vi "Main.vi"() -> ()   [LabVIEW 2019]
doc: "This template is for the Queued Message Handler design pattern.\n\nThe Event Handling Loop generates messages based on user interface actions.\n\nThe Message Handling Loop processes messages generated by the Event Handling Loop, or by other messages. The messages are string values, so new messages can be added easily to the Message Cases case structure in the Message Handling Loop. Each message cluster can also provide an optional value for Message Data, which is a variant that can be converted to whatever message-specific data is required."
uses:
  controls/UI Data.ctl
  support/Message Queue/Enqueue Message (Single).vi
  <vilib>/Utility/error.llb/Error Cluster From Error Code.vi
  <vilib>/ErrorRing/Error Ring.xnode
  support/Message Queue/Message Queue.lvlib
  support/User Event - Stop/User Event - Stop.lvlib
panel:
  in  "Finish":bool
  in  "Restart":bool
  out "Progress":u8(slide) scale=0.0..12.0
  in  "Convert":bool
  out "Tab Control":T1(tab)
  in  "Load File":bool
  in  "Number of Pole Pairs":dbl
  in  "D-Q Transform Angle":dbl
  in  "Phase A Resistance":dbl
  in  "Resistance A unit":enum16{"Ohms", "mOhms", "uOhms"}(ring)
  in  "Phase B Resistance":dbl
  in  "Resistance B unit":enum16{"Ohms", "mOhms", "uOhms"}(ring)
  in  "Phase C Resistance":dbl
  in  "Resistance C unit":enum16{"Ohms", "mOhms", "uOhms"}(ring)
  in  "Direct Current (Id)":dbl[](array[numeric])
  in  "Id unit":enum16{"A", "mA"}(ring)
  in  "Quadratic Current (Iq)":dbl[](array[numeric])
  in  "Iq unit":enum16{"A", "mA"}(ring)
  in  "Direct Inductance (Ld)":dbl[][](array[numeric])
  in  "Ld unit":enum16{"H", "mH", "uH"}(ring)
  in  "Quadratic Inductance (Lq)":dbl[][](array[numeric])
  in  "Lq unit":enum16{"H", "mH", "uH"}(ring)
  in  "Permanent Magnet Flux (Fm)":dbl[][](array[numeric])
  in  "Fm unit":enum16{"Wb", "mWb"}(ring)
  in  "Perm Magnet Flux Scalar":dbl caption="Permanet Magnet Flux (Fm)"
  out "Iq size":i32
  out "Id size":i32
  out "Status":string
  out "Ld":i32[](array[numeric])
  out "Fm":i32[](array[numeric])
  out "Lq":i32[](array[numeric])
  out "JSON File Path":path
  in  "Back":bool
  in  "Next":bool
  # "Step 1: Select the spreadsheet file containing the machine parameters and click Next once it is open."
  # "Step 2: Please fill in the field below with the Number of Poles Pairs OR copy it from the spreadsheet."
  # "Step 3: Please fill in the field below with the D-Q Transform Angle OR copy it from the spreadsheet. Leave it as 0 if you don't have this information."
  # "Step 4: Please fill in the field below with the Phase A Resistance OR copy it from the spreadsheet."
  # "Step 5: Please fill in the field below with the Phase B Resistance OR copy it from the spreadsheet."
  # "Step 6: Please fill in the field below with the Phase C Resistance OR copy it from the spreadsheet."
  # "Step 7: Please fill in the field below with the Current values along the Direct axis of the stator OR copy it from the spreadsheet."
  # "Unit:"
  # "Step 8: Please fill in the field below with the Current values along the Quadratic axis of the stator OR copy it from the spreadsheet."
  # "Unit:"
  # "Step 9: Please fill in the field below with the Direct Inductance OR copy it from the spreadsheet."
  # "Unit:"
  # "Step 10: Please fill in the field below with the Quadratic Inductance OR copy it from the spreadsheet."
  # "Unit:"
  # "Step 11: Please fill in the field below with the Permanent Magnet Flux OR copy it from the spreadsheet. NOTE: Fm parameter is accepted as a scalar or 2D-array."
  # "Unit:"
  # "Step 12: Model converted and saved in the following directory:"
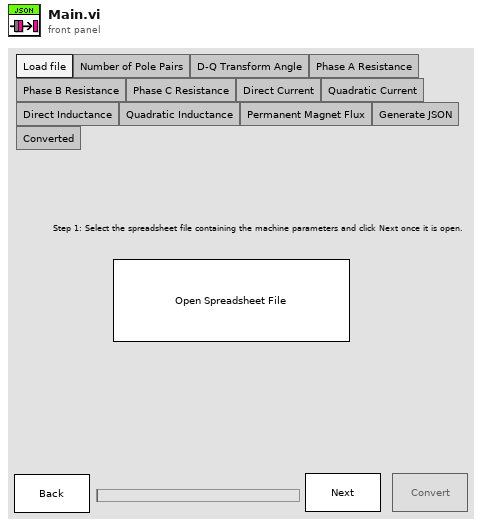
[diagram p1: front panel]
types:
  T1 = enum32{"Load file", "Number of Pole Pairs", "D-Q Transform Angle", "Phase A Resistance", "Phase B Resistance", "Phase C Resistance", "Direct Current", "Quadratic Current", "Direct Inductance", "Quadratic Inductance", "Permanent Magnet Flux", "Generate JSON", "Converted"}
  T2 = typedef "UI Data.ctl" = cluster{"Active tab":u32, "Next ref":refnum<vi>, "Back ref":refnum<vi>, "Convert ref":refnum<vi>, "Restart ref":refnum<vi>, "Finish ref":refnum<vi>, "selected path":path, "VDQ Model":cluster{"PolePairs":dbl, "DqTransformAngleOffset":dbl, "Ra":dbl, "Rb":dbl, "Rc":dbl, "Id_axis":dbl[], "Iq_axis":dbl[], "Ld":dbl[][], "Lq":dbl[][], "Fm":dbl[][]}, "saved path":path, "Scalar Fm ref":refnum<vi>, "2D Fm ref":refnum<vi>, "Current sorted?":cluster{"Id sorted?":bool, "Iq sorted?":bool}}
  T3 = typedef "Message Queue.lvlib/All Message Queues.ctl" = cluster{"UI":refnum<queue>}
  T4 = enum8{"Enabled", "Disabled", "Disabled and Grayed Out"}
  T5 = enum16{"open", "replace", "create", "open or create", "replace or create", "replace or create with confirmation"}
  T6 = cluster{"Id size":i32, "Iq size":i32, "Ld size":i32[], "Lq size":i32[], "FM size":i32[]}
  T7 = cluster{"PolePairs":dbl, "DqTransformAngleOffset":dbl, "Ra":dbl, "Rb":dbl, "Rc":dbl, "Id_axis":dbl[], "Iq_axis":dbl[], "Ld":dbl[][], "Lq":dbl[][], "Fm":dbl[][]}
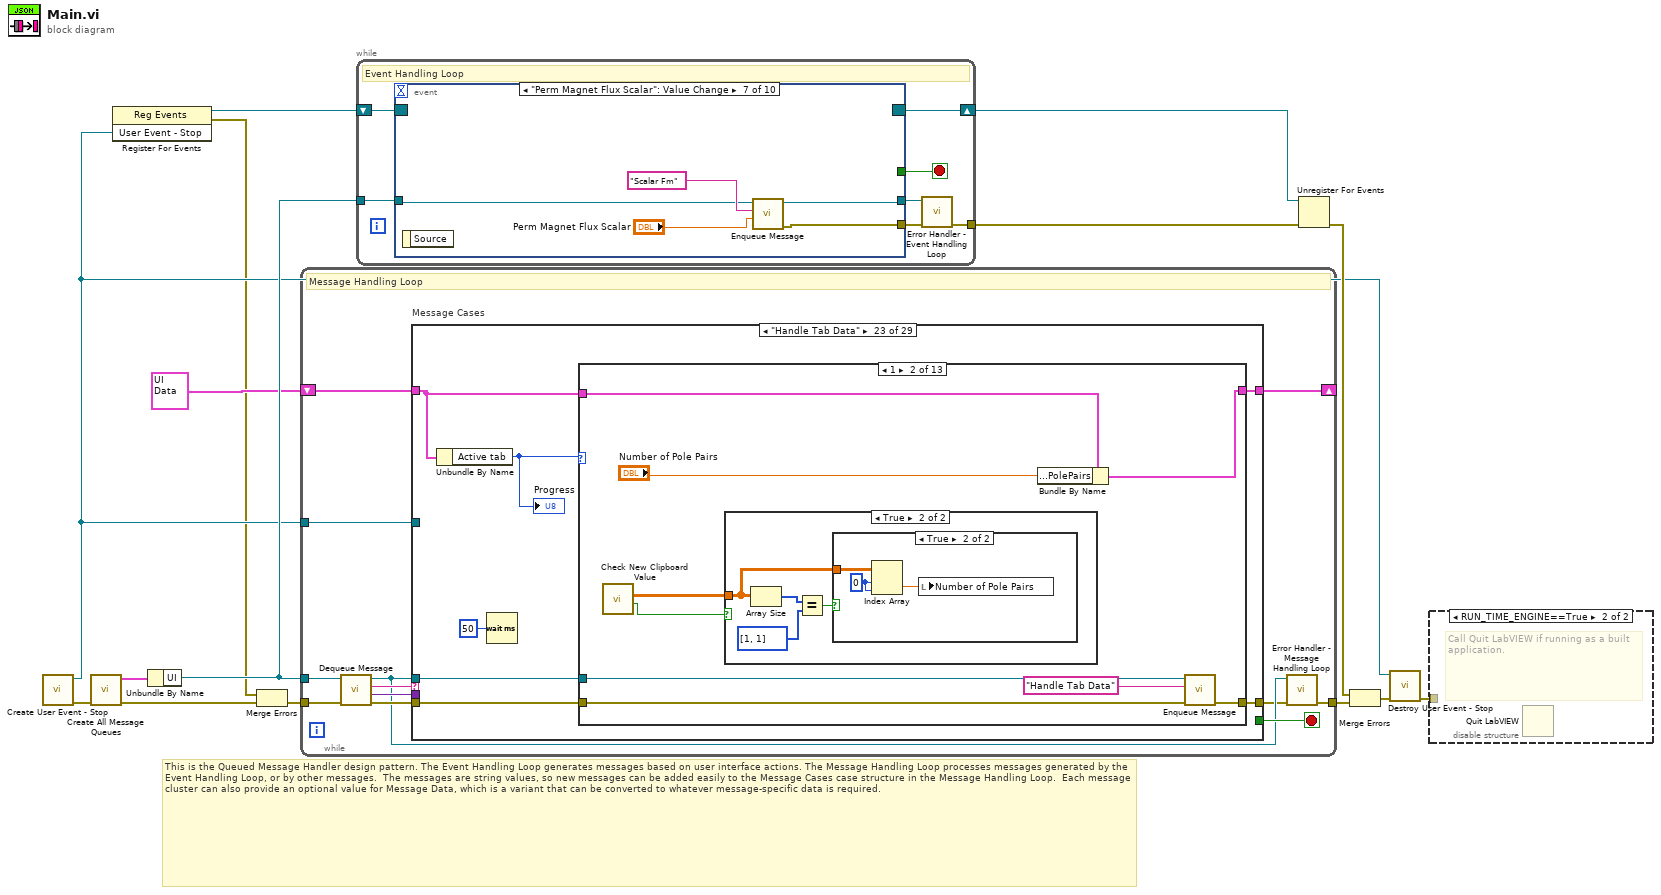
[diagram p0: block diagram]
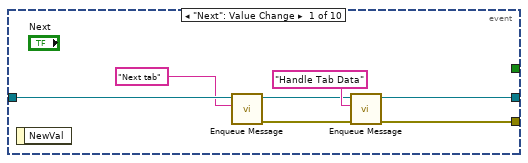
[diagram p3: hidden frame]
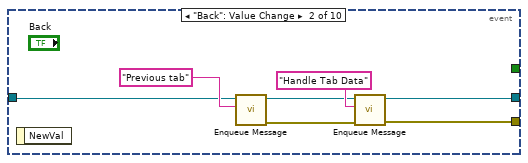
[diagram p4: hidden frame]
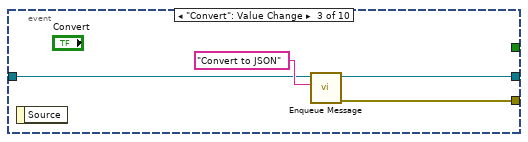
[diagram p5: hidden frame]
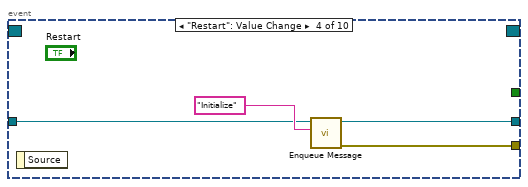
[diagram p6: hidden frame]
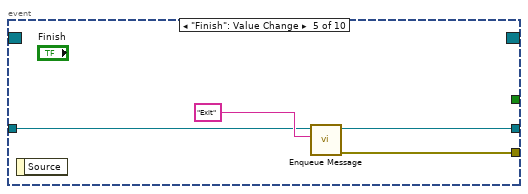
[diagram p7: hidden frame]
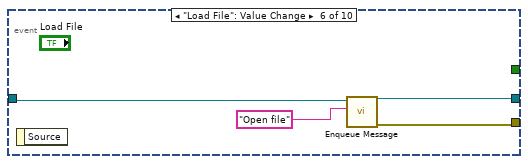
[diagram p8: hidden frame]
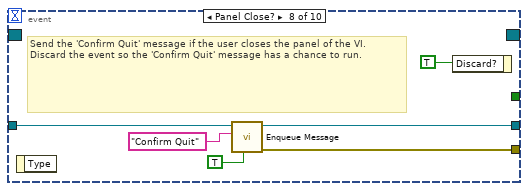
[diagram p9: hidden frame]
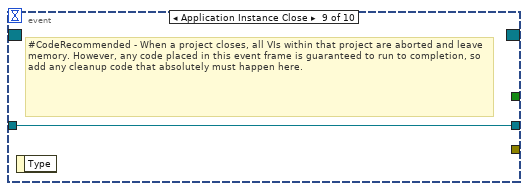
[diagram p10: hidden frame]
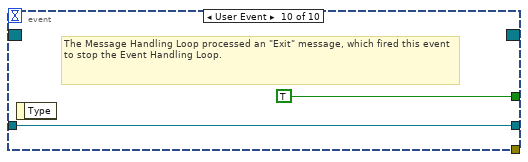
[diagram p11: hidden frame]
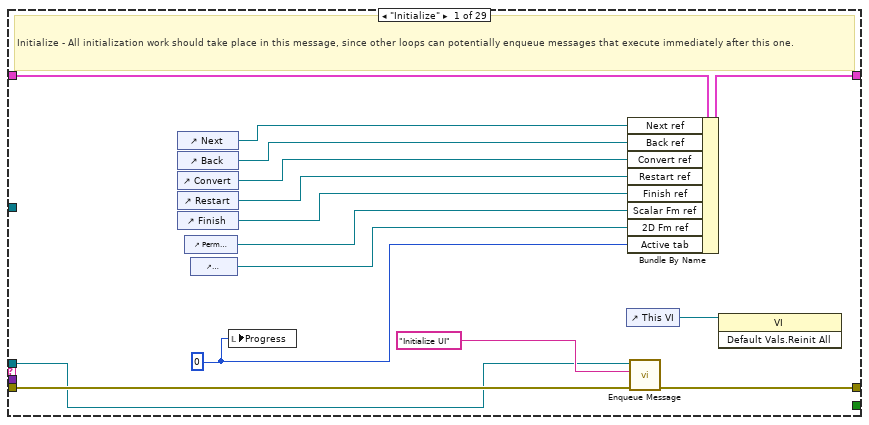
[diagram p12: hidden frame]
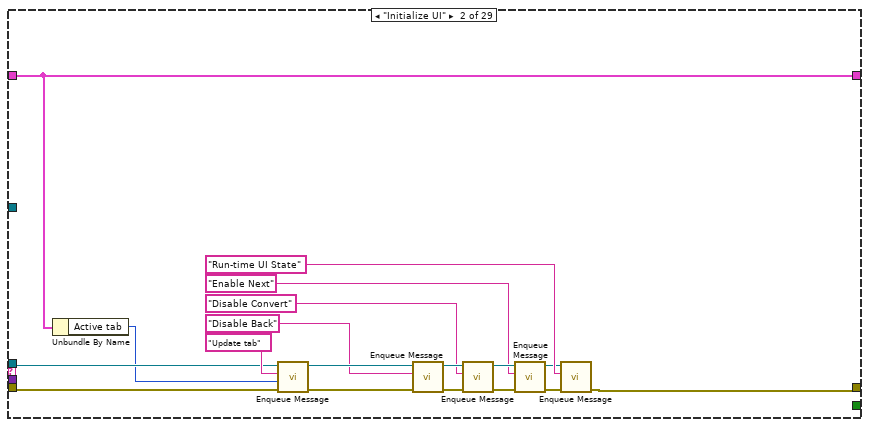
[diagram p13: hidden frame]
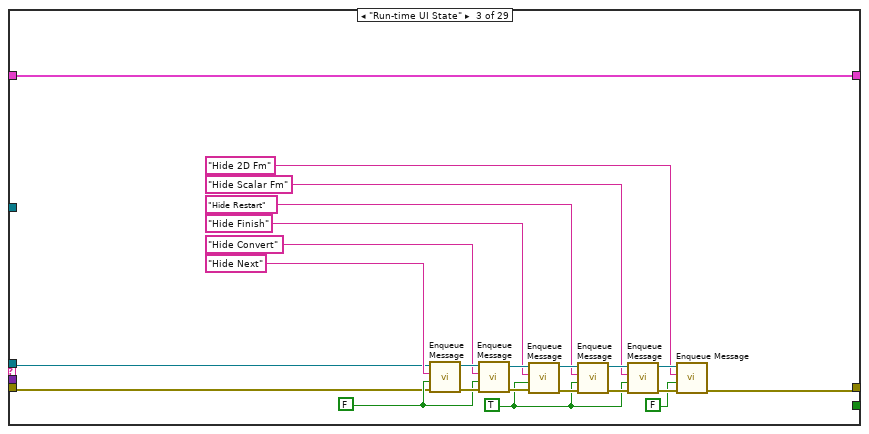
[diagram p14: hidden frame]
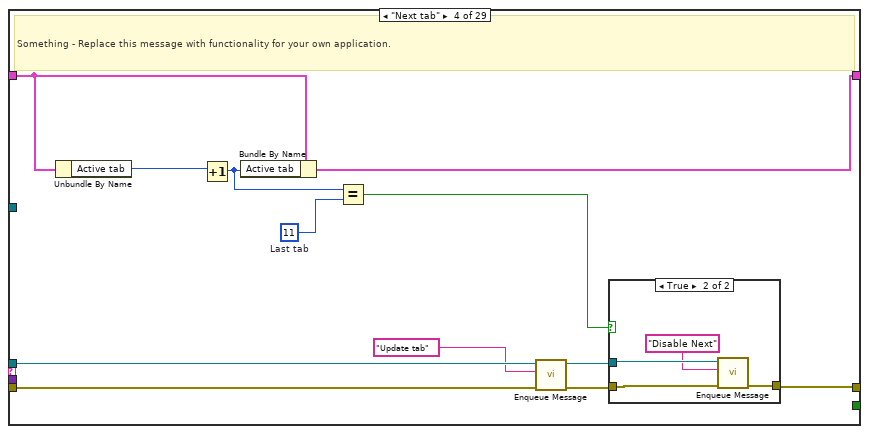
[diagram p15: hidden frame]
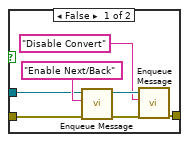
[diagram p16: hidden frame]
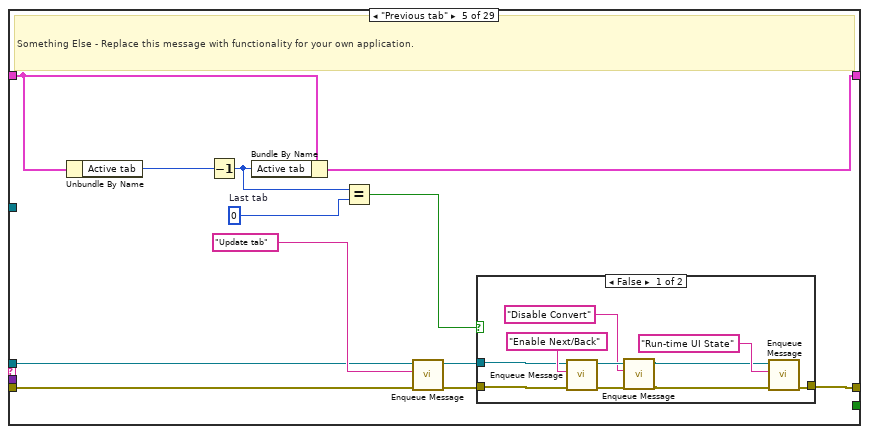
[diagram p17: hidden frame]
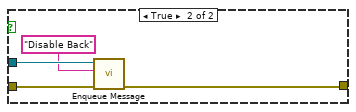
[diagram p18: hidden frame]
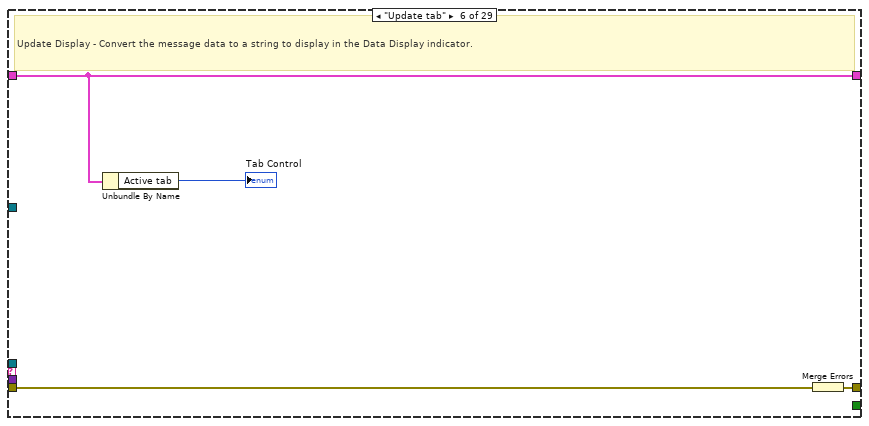
[diagram p19: hidden frame]
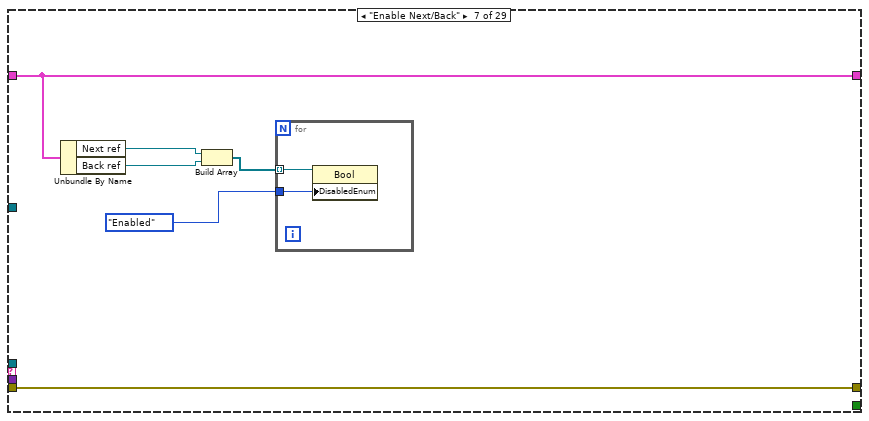
[diagram p20: hidden frame]
diagram:
  # "This is the Queued Message Handler design pattern. The Event Handling Loop generates messages based on user interface actions. The Message Handling Loop processes messages generated by the Event Handling Loop, or by other messages.  The messages are string values, so new messages can be added easily to the Message Cases case structure in the Message Handling Loop.  Each message cluster can also provide an optional value for Message Data, which is a variant that can be converted to whatever message-specific data is required."
  n1 = call "Create User Event - Stop.vi"() -> ("error out"=w11:errorcluster, "User Event - Stop"=w3:refnum<user-event>)  [unwired: 10 in]
  n2 = call "Create All Message Queues.vi"("error in (no error)"=w11) -> ("error out"=w15:errorcluster, "Message Queues out"=w14:T3)  [unwired: 9 in]
  n3 = register-events(w3) -> (reference out=w4:refnum<event-registration>, error out=w1:errorcluster)  [unwired: 2 in]
  n4 = Unbundle By Name(w14) -> ("UI"=w12:refnum<queue>)
  n5 = Merge Errors(w1, w15) -> (w2:errorcluster)
  n6 = while {
    tunnel: w12 -> [w19]
    shift-right: [w26] -> _
    shift-left: T2 {"Active tab"=0, "Next ref"=refnum, "Back ref"=refnum, "Convert ref"=refnum, "Restart ref"=refnum, "Finish ref"=refnum, "selected path"=path "", "VDQ Model"={"PolePairs"=0.0, "DqTransformAngleOffset"=0.0, "Ra"=0.0, "Rb"=0.0, "Rc"=0.0, "Id_axis"=[], "Iq_axis"=[], "Ld"=[], "Lq"=[], "Fm"=[]}, "saved path"=path "", "Scalar Fm ref"=refnum, "2D Fm ref"=refnum, "Current sorted?"={"Id sorted?"=FALSE, "Iq sorted?"=FALSE}} ("Data Cluster") -> [w27]
    tunnel: w3 -> [w24]
    tunnel: w2 -> [w23]
    tunnel: [w17] -> w13
    stop <- w25 stop-if-true
    # "Message Handling Loop"
    n7 = call "Dequeue Message.vi"("error in (no error)"=w23, "Message Queue"=w19) -> ("error out"=w22:errorcluster, "Message Data"=w20:variant, "Message"=w21:string, "dup Message Queue"=w18:refnum<queue>)  [unwired: 6 in]
    n8 = case "Message Cases" shown="\"Handle Tab Data\"" w21 {
      selector: w21 -> [_ _ _ _ _ _ _ _ _ _ _ _ _ _ _ _ _ _ _ _ _ _ _ _ _ _ _ _ w587]
      tunnel: w18 -> [w36 w49 w71 w94 w117 _ _ _ _ _ _ _ _ _ _ _ _ _ w223 _ _ _ w260 w531 _ w568 _ w586 _]
      tunnel: w22 -> [w42 w50 w70 w95 w116 w135 w142 w148 w152 w154 w159 w164 w170 w182 w191 w200 w209 w218 w222 w239 w247 w258 w264 w521 w565 w572 w575 w579 _]
      tunnel: [w31 w43 w66 w84 w108 w136 w142 w148 w152 w153 w158 w163 w172 w183 w192 w201 w210 w219 w224 w239 w246 w248 w265 w543 w559 w570 w573 w582 w588] -> w16
      tunnel: w27 -> [w41 w48 w83 w91 w115 w134 w141 w147 w151 w157 w162 w167 w176 w185 w194 w203 w212 w221 w237 w238 w244 w250 w262 w540 w564 w571 w574 w585 w589]
      tunnel: [w40 w48 w83 w90 w114 w134 w141 w147 w151 w157 w162 w167 w176 w185 w194 w203 w212 w221 w237 w238 w245 w250 w263 w539 w564 w571 w574 w585 w589] -> w26
      tunnel: [_ _ _ _ _ _ _ _ _ _ _ _ _ _ _ _ _ _ _ _ _ _ _ _ _ _ _ TRUE _] -> w25
      tunnel: w20 -> [_ _ _ _ _ _ _ _ _ _ _ _ w169 w179 w188 w197 w206 w215 _ _ _ w257 _ _ w563 _ _ w576 _]
      tunnel: w24 -> [_ _ _ _ _ _ _ _ _ _ _ _ _ _ _ _ _ _ _ _ _ _ _ _ _ _ _ w581 _]
      frame "Initialize" {
        w34 = u32 0
        # "Initialize - All initialization work should take place in this message, since other loops can potentially enqueue messages that execute immediately after this one."
        n9 = control-ref of="Next"() -> (w39:refnum<vi>)
        n10 = control-ref of="Back"() -> (w37:refnum<vi>)
        n11 = control-ref of="Convert"() -> (w35:refnum<vi>)
        n12 = control-ref of="Restart"() -> (w33:refnum<vi>)
        n13 = control-ref of="Finish"() -> (w32:refnum<vi>)
        n14 = control-ref of="Perm Magnet Flux Scalar"() -> (w29:refnum<vi>)
        n15 = control-ref of="Permanent Magnet Flux (Fm)"() -> (w28:refnum<vi>)
        n16 = local write "Progress"(w34) -> ()
        n17 = control-ref of="This VI"() -> (w30:refnum<vi>)
        n18 = Bundle By Name(cluster=w41, "Next ref"=w39, "Back ref"=w37, "Convert ref"=w35, "Restart ref"=w33, "Finish ref"=w32, "Scalar Fm ref"=w29, "2D Fm ref"=w28, "Active tab"=w34) -> (w40:T2)
        n19 = call-poly "Enqueue Message.vi"("error in (no error)"=w42, "Message"="Initialize UI", "Message Queue"=w36) -> ("error out"=w31:errorcluster)  [unwired: 7 in, 1 out]
        n20 = invoke class="VI" method="Default Vals.Reinit All"(reference=w30) -> ()  [unwired: 2 in, 3 out]
      }
      frame "Initialize UI" {
        n21 = Unbundle By Name(w48) -> ("Active tab"=w47:u32)
        n22 = call-poly "Enqueue Message.vi"("error in (no error)"=w50, "Message Data"=w47, "Message"="Update tab", "Message Queue"=w49) -> ("error out"=w60:errorcluster, "dup Message Queue"=w59:refnum<queue>)  [unwired: 6 in]
        n23 = call-poly "Enqueue Message.vi"("error in (no error)"=w60, "Message"="Disable Back", "Message Queue"=w59) -> ("error out"=w58:errorcluster, "dup Message Queue"=w57:refnum<queue>)  [unwired: 7 in]
        n24 = call-poly "Enqueue Message.vi"("error in (no error)"=w58, "Message"="Disable Convert", "Message Queue"=w57) -> ("error out"=w56:errorcluster, "dup Message Queue"=w55:refnum<queue>)  [unwired: 7 in]
        n25 = call-poly "Enqueue Message.vi"("error in (no error)"=w56, "Message"="Enable Next", "Message Queue"=w55) -> ("error out"=w44:errorcluster, "dup Message Queue"=w45:refnum<queue>)  [unwired: 7 in]
        n26 = call-poly "Enqueue Message.vi"("error in (no error)"=w44, "Message"="Run-time UI State", "Message Queue"=w45) -> ("error out"=w43:errorcluster)  [unwired: 7 in, 1 out]
      }
      frame "Run-time UI State" {
        w62 = TRUE
        w72 = FALSE
        n27 = call-poly "Enqueue Message.vi"("error in (no error)"=w70, "Message Data"=w72, "Message"="Hide Next", "Message Queue"=w71) -> ("error out"=w75:errorcluster, "dup Message Queue"=w81:refnum<queue>)  [unwired: 6 in]
        n28 = call-poly "Enqueue Message.vi"("error in (no error)"=w75, "Message Data"=w72, "Message"="Hide Convert", "Message Queue"=w81) -> ("error out"=w74:errorcluster, "dup Message Queue"=w80:refnum<queue>)  [unwired: 6 in]
        n29 = call-poly "Enqueue Message.vi"("error in (no error)"=w74, "Message Data"=w62, "Message"="Hide Finish", "Message Queue"=w80) -> ("error out"=w73:errorcluster, "dup Message Queue"=w79:refnum<queue>)  [unwired: 6 in]
        n30 = call-poly "Enqueue Message.vi"("error in (no error)"=w73, "Message Data"=w62, "Message"="Hide Restart", "Message Queue"=w79) -> ("error out"=w67:errorcluster, "dup Message Queue"=w65:refnum<queue>)  [unwired: 6 in]
        n31 = call-poly "Enqueue Message.vi"("error in (no error)"=w67, "Message Data"=w62, "Message"="Hide Scalar Fm", "Message Queue"=w65) -> ("error out"=w69:errorcluster, "dup Message Queue"=w68:refnum<queue>)  [unwired: 6 in]
        n32 = call-poly "Enqueue Message.vi"("error in (no error)"=w69, "Message Data"=FALSE, "Message"="Hide 2D Fm", "Message Queue"=w68) -> ("error out"=w66:errorcluster)  [unwired: 6 in, 1 out]
      }
      frame "Next tab" {
        w89 = u32 11  # Last tab
        # "Something - Replace this message with functionality for your own application."
        n33 = Unbundle By Name(w91) -> ("Active tab"=w92:u32)
        n34 = Increment(x=w92) -> (x+1=w88:u32)
        n35 = Bundle By Name(cluster=w91, "Active tab"=w88) -> (w90:T2)
        n36 = Equal?(x=w88, y=w89) -> (x = y?=w87:bool)
        n37 = call-poly "Enqueue Message.vi"("error in (no error)"=w95, "Message"="Update tab", "Message Queue"=w94) -> ("error out"=w86:errorcluster, "dup Message Queue"=w85:refnum<queue>)  [unwired: 7 in]
        n38 = case shown="True" w87 {
          tunnel: w86 -> [w101 w106]
          tunnel: w85 -> [w100 w104]
          tunnel: [w98 w105] -> w84
          frame False {
            n39 = call-poly "Enqueue Message.vi"("error in (no error)"=w101, "Message"="Enable Next/Back", "Message Queue"=w100) -> ("error out"=w99:errorcluster, "dup Message Queue"=w97:refnum<queue>)  [unwired: 7 in]
            n40 = call-poly "Enqueue Message.vi"("error in (no error)"=w99, "Message"="Disable Convert", "Message Queue"=w97) -> ("error out"=w98:errorcluster)  [unwired: 7 in, 1 out]
          }
          frame True {
            n41 = call-poly "Enqueue Message.vi"("error in (no error)"=w106, "Message"="Disable Next", "Message Queue"=w104) -> ("error out"=w105:errorcluster)  [unwired: 7 in, 1 out]
          }
        }
      }
      frame "Previous tab" {
        w112 = u32 0  # Last tab
        # "Something Else - Replace this message with functionality for your own application."
        n42 = Unbundle By Name(w115) -> ("Active tab"=w113:u32)
        n43 = Decrement(x=w113) -> (x-1=w107:u32)
        n44 = Bundle By Name(cluster=w115, "Active tab"=w107) -> (w114:T2)
        n45 = Equal?(x=w107, y=w112) -> (x = y?=w111:bool)
        n46 = call-poly "Enqueue Message.vi"("error in (no error)"=w116, "Message"="Update tab", "Message Queue"=w117) -> ("error out"=w110:errorcluster, "dup Message Queue"=w109:refnum<queue>)  [unwired: 7 in]
        n47 = case shown="False" w111 {
          tunnel: w110 -> [w124 w132]
          tunnel: w109 -> [w123 w131]
          tunnel: [w119 w129] -> w108
          frame False {
            n48 = call-poly "Enqueue Message.vi"("error in (no error)"=w124, "Message"="Enable Next/Back", "Message Queue"=w123) -> ("error out"=w127:errorcluster, "dup Message Queue"=w126:refnum<queue>)  [unwired: 7 in]
            n49 = call-poly "Enqueue Message.vi"("error in (no error)"=w127, "Message"="Disable Convert", "Message Queue"=w126) -> ("error out"=w120:errorcluster, "dup Message Queue"=w121:refnum<queue>)  [unwired: 7 in]
            n50 = call-poly "Enqueue Message.vi"("error in (no error)"=w120, "Message"="Run-time UI State", "Message Queue"=w121) -> ("error out"=w119:errorcluster)  [unwired: 7 in, 1 out]
          }
          frame True {
            n51 = call-poly "Enqueue Message.vi"("error in (no error)"=w132, "Message"="Disable Back", "Message Queue"=w131) -> ("error out"=w129:errorcluster)  [unwired: 7 in, 1 out]
          }
        }
      }
      frame "Update tab" {
        # "Update Display - Convert the message data to a string to display in the Data Display indicator."
        n52 = Unbundle By Name(w134) -> ("Active tab"=→"Tab Control":u32)
        n53 = Merge Errors(w135) -> (w136:errorcluster)
      }
      frame "Enable Next/Back" {
        n54 = Unbundle By Name(w141) -> ("Next ref"=w140:refnum<vi>, "Back ref"=w139:refnum<vi>)
        n55 = Build Array(w140, w139) -> (w138:refnum<vi>[])
        n56 = for {
          tunnel: w138 -> [w144] mode=indexing
          tunnel: T4."Enabled" ("Disabled") -> [w143]
          n57 = property class="Bool"(reference=w144, "DisabledEnum"=w143) -> ()  [unwired: 1 in, 2 out]
        }
      }
      frame "Enable Convert" {
        n58 = Unbundle By Name(w147) -> ("Convert ref"=w145:refnum<vi>)
        n59 = property class="Bool"(reference=w145, "DisabledEnum"=T4."Enabled" ("Disabled")) -> ()  [unwired: 1 in, 2 out]
      }
      frame "Enable Next" {
        n60 = Unbundle By Name(w151) -> ("Next ref"=w149:refnum<vi>)
        n61 = property class="Bool"(reference=w149, "DisabledEnum"=T4."Enabled" ("Disabled")) -> ()  [unwired: 1 in, 2 out]
      }
      frame "Disable Next" {
        n62 = Unbundle By Name(w157) -> ("Next ref"=w156:refnum<vi>)
        n63 = property class="Bool"(reference=w156, error in=w154, "DisabledEnum"=T4."Disabled and Grayed Out" ("Disabled")) -> (error out=w153:errorcluster)  [unwired: 1 out]
      }
      frame "Disable Back" {
        n64 = Unbundle By Name(w162) -> ("Back ref"=w161:refnum<vi>)
        n65 = property class="Bool"(reference=w161, error in=w159, "DisabledEnum"=T4."Disabled and Grayed Out" ("Disabled")) -> (error out=w158:errorcluster)  [unwired: 1 out]
      }
      frame "Disable Convert" {
        n66 = Unbundle By Name(w167) -> ("Convert ref"=w166:refnum<vi>)
        n67 = property class="Bool"(reference=w166, error in=w164, "DisabledEnum"=T4."Disabled and Grayed Out" ("Disabled")) -> (error out=w163:errorcluster)  [unwired: 1 out]
      }
      frame "Hide Next" {
        n68 = Variant To Data(error in=w170, type=FALSE ("Visible"), Variant=w169) -> (data=w173:bool, error out=w175:errorcluster)
        n69 = Unbundle By Name(w176) -> ("Next ref"=w171:refnum<vi>)
        n70 = Not(x=w173) -> (.not. x?=w168:bool)
        n71 = property class="Bool"(reference=w171, error in=w175, "Visible"=w168) -> (error out=w172:errorcluster)  [unwired: 1 out]
      }
      frame "Hide Convert" {
        n72 = Variant To Data(error in=w182, type=FALSE ("Visible"), Variant=w179) -> (data=w178:bool, error out=w181:errorcluster)
        n73 = Unbundle By Name(w185) -> ("Convert ref"=w184:refnum<vi>)
        n74 = Not(x=w178) -> (.not. x?=w177:bool)
        n75 = property class="Bool"(reference=w184, error in=w181, "Visible"=w177) -> (error out=w183:errorcluster)  [unwired: 1 out]
      }
      frame "Hide Restart" {
        n76 = Variant To Data(error in=w191, type=FALSE ("Visible"), Variant=w188) -> (data=w187:bool, error out=w190:errorcluster)
        n77 = Unbundle By Name(w194) -> ("Restart ref"=w193:refnum<vi>)
        n78 = Not(x=w187) -> (.not. x?=w186:bool)
        n79 = property class="Bool"(reference=w193, error in=w190, "Visible"=w186) -> (error out=w192:errorcluster)  [unwired: 1 out]
      }
      frame "Hide Scalar Fm" {
        n80 = Variant To Data(error in=w200, type=FALSE ("Visible"), Variant=w197) -> (data=w196:bool, error out=w199:errorcluster)
        n81 = Unbundle By Name(w203) -> ("Scalar Fm ref"=w202:refnum<vi>)
        n82 = Not(x=w196) -> (.not. x?=w195:bool)
        n83 = property class="DigNum (strict)"(reference=w202, error in=w199, "Visible"=w195) -> (error out=w201:errorcluster)  [unwired: 1 out]
      }
      frame "Hide 2D Fm" {
        n84 = Variant To Data(error in=w209, type=FALSE ("Visible"), Variant=w206) -> (data=w205:bool, error out=w208:errorcluster)
        n85 = Unbundle By Name(w212) -> ("2D Fm ref"=w211:refnum<vi>)
        n86 = Not(x=w205) -> (.not. x?=w204:bool)
        n87 = property class="Arr (strict)"(reference=w211, error in=w208, "Visible"=w204) -> (error out=w210:errorcluster)  [unwired: 1 out]
      }
      frame "Hide Finish" {
        n88 = Variant To Data(error in=w218, type=FALSE ("Visible"), Variant=w215) -> (data=w214:bool, error out=w217:errorcluster)
        n89 = Unbundle By Name(w221) -> ("Finish ref"=w220:refnum<vi>)
        n90 = Not(x=w214) -> (.not. x?=w213:bool)
        n91 = property class="Bool"(reference=w220, error in=w217, "Visible"=w213) -> (error out=w219:errorcluster)  [unwired: 1 out]
      }
      frame "Final UI State" {
        w225 = FALSE
        w226 = TRUE
        n92 = call-poly "Enqueue Message.vi"("error in (no error)"=w222, "Message Data"=w226, "Message"="Hide Next", "Message Queue"=w223) -> ("error out"=w229:errorcluster, "dup Message Queue"=w235:refnum<queue>)  [unwired: 6 in]
        n93 = call-poly "Enqueue Message.vi"("error in (no error)"=w229, "Message Data"=w226, "Message"="Hide Convert", "Message Queue"=w235) -> ("error out"=w228:errorcluster, "dup Message Queue"=w234:refnum<queue>)  [unwired: 6 in]
        n94 = call-poly "Enqueue Message.vi"("error in (no error)"=w228, "Message Data"=w225, "Message"="Hide Finish", "Message Queue"=w234) -> ("error out"=w227:errorcluster, "dup Message Queue"=w233:refnum<queue>)  [unwired: 6 in]
        n95 = call-poly "Enqueue Message.vi"("error in (no error)"=w227, "Message Data"=w225, "Message"="Hide Restart", "Message Queue"=w233) -> ("error out"=w224:errorcluster)  [unwired: 6 in, 1 out]
      }
      frame "-----------------" {
      }
      frame "Open file" {
        n96 = call "File Dialog"("error in"=w247) -> ("selected path"=w243:path, "error out"=w242:errorcluster)  [unwired: 11 in, 2 out]
        n97 = call <vilib>:"Clear Errors.vi"("error in (no error)"=w242, "specific error code to clear (0: all)"=43) -> ("error out"=w240:errorcluster)  [unwired: 4 in, 1 out]
        n98 = call <vilib>:"Open a Document on Disk.vi"("error in (no error)"=w240, "document path"=w243) -> ("error out"=w246:errorcluster)  [unwired: 5 in]
        n99 = Bundle By Name(cluster=w244, "selected path"=w243) -> (w245:T2)
      }
      frame "Scalar Fm" {
        n100 = Variant To Data(error in=w258, type=0.0, Variant=w257) -> (data=w251:dbl, error out=w248:errorcluster)
        n101 = Unbundle By Name(w250) -> ("VDQ Model.Ld"=w252:dbl[][])
        n102 = Array Size(array=w252) -> (size(s)=w255:i32[])
        n103 = Index Array(array=w255) -> (element #1=w254:i32, element #2=w253:i32)  [unwired: 2 in]
        n104 = Initialize Array(w251, w254, w253) -> (w249:dbl[][])
        n105 = local write "Permanent Magnet Flux (Fm)"(w249) -> ()
      }
      frame "Handle Tab Data" {
        n106 = Unbundle By Name(w262) -> ("Active tab"=w259:u32)
        "Progress" <- w259
        n107 = Wait (ms)(milliseconds to wait=u32 50) -> ()  [unwired: 1 out]
        n108 = case shown="1" w259 {
          tunnel: [w267 w270 w288 w303 w322 w340 w360 w385 w410 w436 w461 w487 w517] -> w265
          tunnel: w264 -> [w267 w271 w289 w305 w323 w341 w359 w384 w409 w435 w462 w497 w518]
          tunnel: [w266 w275 w291 w307 w325 w343 w364 w388 w413 w438 w464 w499 w515] -> w263
          tunnel: w262 -> [w266 w276 w292 w308 w326 w344 w365 w389 w404 w430 w456 w499 w515]
          tunnel: w260 -> [_ w269 w287 w304 w321 w339 w358 w383 w408 w434 w460 w496 w516]
          frame 0, Default {
          }
          frame 1 {
            n109 = call "Check New Clipboard Value.vi"() -> ("New Value?"=w272:bool, "Values"=w273:dbl[][])  [unwired: 9 in, 1 out]
            n110 = case shown="True" w272 {
              tunnel: w273 -> [_ w277]
              frame False {
              }
              frame True {
                n111 = Array Size(array=w277) -> (size(s)=w280:i32[])
                n112 = Equal?(x=w280, y=i32[] [1, 1]) -> (x = y?=w278:bool)
                n113 = case shown="True" w278 {
                  tunnel: w277 -> [_ w283]
                  frame False {
                  }
                  frame True {
                    w282 = 0 ("index (row)")
                    n114 = Index Array(array=w283, index (row)=w282, index (col)=w282) -> (element=w281:dbl)
                    n115 = local write "Number of Pole Pairs"(w281) -> ()
                  }
                }
              }
            }
            n116 = Bundle By Name(cluster=w276, "VDQ Model.PolePairs"="Number of Pole Pairs") -> (w275:T2)
            n117 = call-poly "Enqueue Message.vi"("error in (no error)"=w271, "Message"="Handle Tab Data", "Message Queue"=w269) -> ("error out"=w270:errorcluster)  [unwired: 7 in, 1 out]
          }
          frame 2 {
            n118 = call "Check New Clipboard Value.vi"() -> ("New Value?"=w285:bool, "Values"=w286:dbl[][])  [unwired: 9 in, 1 out]
            n119 = case shown="True" w285 {
              tunnel: w286 -> [_ w293]
              frame False {
              }
              frame True {
                n120 = Array Size(array=w293) -> (size(s)=w296:i32[])
                n121 = Equal?(x=w296, y=i32[] [1, 1]) -> (x = y?=w294:bool)
                n122 = case shown="True" w294 {
                  tunnel: w293 -> [_ w299]
                  frame False {
                  }
                  frame True {
                    w298 = 0 ("index (row)")
                    n123 = Index Array(array=w299, index (row)=w298, index (col)=w298) -> (element=w297:dbl)
                    n124 = local write "D-Q Transform Angle"(w297) -> ()
                  }
                }
              }
            }
            n125 = Bundle By Name(cluster=w292, "VDQ Model.DqTransformAngleOffset"="D-Q Transform Angle") -> (w291:T2)
            n126 = call-poly "Enqueue Message.vi"("error in (no error)"=w289, "Message"="Handle Tab Data", "Message Queue"=w287) -> ("error out"=w288:errorcluster)  [unwired: 7 in, 1 out]
          }
          frame 3 {
            n127 = call "Check New Clipboard Value.vi"() -> ("New Value?"=w310:bool, "Values"=w309:dbl[][])  [unwired: 9 in, 1 out]
            n128 = case shown="True" w310 {
              tunnel: w309 -> [_ w311]
              frame False {
              }
              frame True {
                n129 = Array Size(array=w311) -> (size(s)=w314:i32[])
                n130 = Equal?(x=w314, y=i32[] [1, 1]) -> (x = y?=w312:bool)
                n131 = case shown="True" w312 {
                  tunnel: w311 -> [_ w317]
                  frame False {
                  }
                  frame True {
                    w316 = 0 ("index (row)")
                    n132 = Index Array(array=w317, index (row)=w316, index (col)=w316) -> (element=w315:dbl)
                    n133 = local write "Phase A Resistance"(w315) -> ()
                  }
                }
              }
            }
            n134 = call "Convert Unit.vi"("Data in"="Phase A Resistance", "unit"="Resistance A unit") -> ("Data out"=w302:dbl)  [unwired: 7 in]
            n135 = local write "Phase B Resistance"("Phase A Resistance") -> ()
            n136 = local write "Phase C Resistance"("Phase A Resistance") -> ()
            n137 = Bundle By Name(cluster=w308, "VDQ Model.Ra"=w302) -> (w307:T2)
            n138 = local write "Resistance C unit"("Resistance A unit") -> ()
            n139 = local write "Resistance B unit"("Resistance A unit") -> ()
            n140 = call-poly "Enqueue Message.vi"("error in (no error)"=w305, "Message"="Handle Tab Data", "Message Queue"=w304) -> ("error out"=w303:errorcluster)  [unwired: 7 in, 1 out]
          }
          frame 4 {
            n141 = call "Check New Clipboard Value.vi"() -> ("New Value?"=w328:bool, "Values"=w327:dbl[][])  [unwired: 9 in, 1 out]
            n142 = case shown="True" w328 {
              tunnel: w327 -> [_ w329]
              frame False {
              }
              frame True {
                n143 = Array Size(array=w329) -> (size(s)=w332:i32[])
                n144 = Equal?(x=w332, y=i32[] [1, 1]) -> (x = y?=w330:bool)
                n145 = case shown="True" w330 {
                  tunnel: w329 -> [_ w335]
                  frame False {
                  }
                  frame True {
                    w334 = 0 ("index (row)")
                    n146 = Index Array(array=w335, index (row)=w334, index (col)=w334) -> (element=w333:dbl)
                    n147 = local write "Phase B Resistance"(w333) -> ()
                  }
                }
              }
            }
            n148 = call "Convert Unit.vi"("Data in"="Phase B Resistance", "unit"="Resistance B unit") -> ("Data out"=w320:dbl)  [unwired: 7 in]
            n149 = local write "Phase C Resistance"("Phase B Resistance") -> ()
            n150 = Bundle By Name(cluster=w326, "VDQ Model.Rb"=w320) -> (w325:T2)
            n151 = local write "Resistance C unit"("Resistance B unit") -> ()
            n152 = call-poly "Enqueue Message.vi"("error in (no error)"=w323, "Message"="Handle Tab Data", "Message Queue"=w321) -> ("error out"=w322:errorcluster)  [unwired: 7 in, 1 out]
          }
          frame 5 {
            n153 = call "Check New Clipboard Value.vi"() -> ("New Value?"=w346:bool, "Values"=w345:dbl[][])  [unwired: 9 in, 1 out]
            n154 = case shown="True" w346 {
              tunnel: w345 -> [_ w347]
              frame False {
              }
              frame True {
                n155 = Array Size(array=w347) -> (size(s)=w350:i32[])
                n156 = Equal?(x=w350, y=i32[] [1, 1]) -> (x = y?=w348:bool)
                n157 = case shown="True" w348 {
                  tunnel: w347 -> [_ w353]
                  frame False {
                  }
                  frame True {
                    w352 = 0 ("index (row)")
                    n158 = Index Array(array=w353, index (row)=w352, index (col)=w352) -> (element=w351:dbl)
                    n159 = local write "Phase C Resistance"(w351) -> ()
                  }
                }
              }
            }
            n160 = call "Convert Unit.vi"("Data in"="Phase C Resistance", "unit"="Resistance C unit") -> ("Data out"=w337:dbl)  [unwired: 7 in]
            n161 = Bundle By Name(cluster=w344, "VDQ Model.Rc"=w337) -> (w343:T2)
            n162 = call-poly "Enqueue Message.vi"("error in (no error)"=w341, "Message"="Handle Tab Data", "Message Queue"=w339) -> ("error out"=w340:errorcluster)  [unwired: 7 in, 1 out]
          }
          frame 6 {
            n163 = call "Check New Clipboard Value.vi"() -> ("New Value?"=w362:bool, "Values"=w363:dbl[][])  [unwired: 9 in, 1 out]
            n164 = case shown="True" w362 {
              tunnel: w363 -> [_ w370]
              tunnel: [FALSE ("Sorted?") w367] -> w354
              frame False {
              }
              frame True {
                n165 = call "is a 1D-array"("Values"=w370) -> ("Number of elements"=w368:i32, "1D-Array?"=w369:bool)  [unwired: 1 in]
                n166 = case shown="True" w369 {
                  tunnel: w370 -> [_ w377]
                  tunnel: w368 -> [_ w376]
                  tunnel: [FALSE ("Sorted?") w372] -> w367
                  frame False {
                  }
                  frame True {
                    n167 = Reshape Array(w377, w376) -> (w375:dbl[])
                    n168 = call "Sort Current in Ascending Order.vi"("Current Array in"=w375) -> ("Sorted?"=w372:bool, "Current Array out"=w374:dbl[], "Not ascending/descending order?"=w373:bool)  [unwired: 7 in]
                    n169 = case shown="True" w373 {
                      frame False {
                      }
                      frame True {
                        n170 = One Button Dialog(message="The current array should be arranged in ascending or descending order") -> ()  [unwired: 1 in, 1 out]
                      }
                    }
                    n171 = local write "Direct Current (Id)"(w374) -> ()
                  }
                }
              }
            }
            n172 = call "Convert Unit (1D-Array).vi"("Data in"="Direct Current (Id)", "unit"="Id unit") -> ("Data out"=w355:dbl[])  [unwired: 7 in]
            n173 = Bundle By Name(cluster=w365, "VDQ Model.Id_axis"=w355, "Current sorted?.Id sorted?"=w354) -> (w364:T2)
            n174 = call-poly "Enqueue Message.vi"("error in (no error)"=w359, "Message"="Handle Tab Data", "Message Queue"=w358) -> ("error out"=w360:errorcluster)  [unwired: 7 in, 1 out]
          }
          frame 7 {
            n175 = call "Check New Clipboard Value.vi"() -> ("New Value?"=w387:bool, "Values"=w390:dbl[][])  [unwired: 9 in, 1 out]
            n176 = case shown="True" w387 {
              tunnel: w390 -> [_ w395]
              tunnel: [FALSE ("Sorted?") w392] -> w379
              frame False {
              }
              frame True {
                n177 = call "is a 1D-array"("Values"=w395) -> ("Number of elements"=w393:i32, "1D-Array?"=w394:bool)  [unwired: 1 in]
                n178 = case shown="True" w394 {
                  tunnel: w395 -> [_ w402]
                  tunnel: w393 -> [_ w401]
                  tunnel: [FALSE ("Sorted?") w397] -> w392
                  frame False {
                  }
                  frame True {
                    n179 = Reshape Array(w402, w401) -> (w398:dbl[])
                    n180 = call "Sort Current in Ascending Order.vi"("Current Array in"=w398) -> ("Sorted?"=w397:bool, "Current Array out"=w400:dbl[], "Not ascending/descending order?"=w399:bool)  [unwired: 7 in]
                    n181 = local write "Quadratic Current (Iq)"(w400) -> ()
                    n182 = case shown="True" w399 {
                      frame False {
                      }
                      frame True {
                        n183 = One Button Dialog(message="The current array should be arranged in ascending or descending order") -> ()  [unwired: 1 in, 1 out]
                      }
                    }
                  }
                }
              }
            }
            n184 = call "Convert Unit (1D-Array).vi"("Data in"="Quadratic Current (Iq)", "unit"="Iq unit") -> ("Data out"=w381:dbl[])  [unwired: 7 in]
            n185 = Bundle By Name(cluster=w389, "VDQ Model.Iq_axis"=w381, "Current sorted?.Iq sorted?"=w379) -> (w388:T2)
            n186 = call-poly "Enqueue Message.vi"("error in (no error)"=w384, "Message"="Handle Tab Data", "Message Queue"=w383) -> ("error out"=w385:errorcluster)  [unwired: 7 in, 1 out]
          }
          frame 8 {
            n187 = call "Check New Clipboard Value.vi"() -> ("New Value?"=w412:bool, "Values"=w414:dbl[][])  [unwired: 9 in, 1 out]
            n188 = case shown="True" w412 {
              tunnel: w414 -> [_ w416]
              tunnel: w404 -> [_ w422]
              frame False {
              }
              frame True {
                n189 = Unbundle By Name(w422) -> ("Current sorted?"=w423:cluster{"Id sorted?":bool, "Iq sorted?":bool})
                n190 = call "is a 2D-array.vi"("Values"=w416) -> ("2D-Array?"=w419:bool)
                n191 = Array Size(array=w416) -> (size(s)=w421:i32[])
                n192 = Equal?(x=w421, y=i32[] [1, 1]) -> (x = y?=w420:bool)
                n193 = Build Array(w419, w420) -> (w418:bool[])
                n194 = Boolean Array To Number(Boolean array=w418) -> (number=w415:u32)
                n195 = case shown="2" w415 {
                  tunnel: w416 -> [_ w425 w429]
                  tunnel: w423 -> [_ w426 _]
                  tunnel: w422 -> [_ _ w428]
                  frame 0, Default {
                  }
                  frame 1 {
                    n196 = call "Sort Inductance Matrix.vi"("Current sorted?"=w426, "Inductance Matrix in"=w425) -> ("Inductance Matrix out"=w424:dbl[][])  [unwired: 2 in]
                    n197 = local write "Direct Inductance (Ld)"(w424) -> ()
                  }
                  frame 2 {
                    n198 = call "Convert Fm to 2D array.vi"("Data in"=w429, "Data Cluster"=w428) -> ("Data out"=w427:dbl[][])  [unwired: 7 in, 1 out]
                    n199 = local write "Direct Inductance (Ld)"(w427) -> ()
                  }
                }
              }
            }
            n200 = call "Convert Unit (2D-Array).vi"("Data in"="Direct Inductance (Ld)", "unit"="Ld unit") -> ("Data out"=w406:dbl[][])  [unwired: 7 in]
            n201 = Bundle By Name(cluster=w404, "VDQ Model.Ld"=w406) -> (w413:T2)
            n202 = call-poly "Enqueue Message.vi"("error in (no error)"=w409, "Message"="Handle Tab Data", "Message Queue"=w408) -> ("error out"=w410:errorcluster)  [unwired: 7 in, 1 out]
          }
          frame 9 {
            n203 = call "Check New Clipboard Value.vi"() -> ("New Value?"=w439:bool, "Values"=w440:dbl[][])  [unwired: 9 in, 1 out]
            n204 = case shown="True" w439 {
              tunnel: w440 -> [_ w444]
              tunnel: w430 -> [_ w441]
              frame False {
              }
              frame True {
                n205 = Unbundle By Name(w441) -> ("Current sorted?"=w449:cluster{"Id sorted?":bool, "Iq sorted?":bool})
                n206 = call "is a 2D-array.vi"("Values"=w444) -> ("2D-Array?"=w446:bool)
                n207 = Array Size(array=w444) -> (size(s)=w448:i32[])
                n208 = Equal?(x=w448, y=i32[] [1, 1]) -> (x = y?=w447:bool)
                n209 = Build Array(w446, w447) -> (w445:bool[])
                n210 = Boolean Array To Number(Boolean array=w445) -> (number=w443:u32)
                n211 = case shown="2" w443 {
                  tunnel: w444 -> [_ w452 w455]
                  tunnel: w449 -> [_ w450 _]
                  tunnel: w441 -> [_ _ w454]
                  frame 0, Default {
                  }
                  frame 1 {
                    n212 = call "Sort Inductance Matrix.vi"("Current sorted?"=w450, "Inductance Matrix in"=w452) -> ("Inductance Matrix out"=w451:dbl[][])  [unwired: 2 in]
                    n213 = local write "Quadratic Inductance (Lq)"(w451) -> ()
                  }
                  frame 2 {
                    n214 = call "Convert Fm to 2D array.vi"("Data in"=w455, "Data Cluster"=w454) -> ("Data out"=w453:dbl[][])  [unwired: 7 in, 1 out]
                    n215 = local write "Quadratic Inductance (Lq)"(w453) -> ()
                  }
                }
              }
            }
            n216 = call "Convert Unit (2D-Array).vi"("Data in"="Quadratic Inductance (Lq)", "unit"="Lq unit") -> ("Data out"=w432:dbl[][])  [unwired: 7 in]
            n217 = Bundle By Name(cluster=w430, "VDQ Model.Lq"=w432) -> (w438:T2)
            n218 = call-poly "Enqueue Message.vi"("error in (no error)"=w435, "Message"="Handle Tab Data", "Message Queue"=w434) -> ("error out"=w436:errorcluster)  [unwired: 7 in, 1 out]
          }
          frame 10 {
            n219 = call "Check New Clipboard Value.vi"() -> ("New Value?"=w465:bool, "Values"=w466:dbl[][])  [unwired: 9 in, 1 out]
            n220 = case shown="True" w465 {
              tunnel: w466 -> [_ w473]
              tunnel: w456 -> [_ w468]
              frame False {
              }
              frame True {
                n221 = call "is a 2D-array.vi"("Values"=w473) -> ("2D-Array?"=w471:bool)
                n222 = Array Size(array=w473) -> (size(s)=w475:i32[])
                n223 = Unbundle By Name(w468) -> ("Current sorted?"=w467:cluster{"Id sorted?":bool, "Iq sorted?":bool})
                n224 = Equal?(x=w475, y=i32[] [1, 1]) -> (x = y?=w472:bool)
                n225 = Build Array(w471, w472) -> (w470:bool[])
                n226 = Boolean Array To Number(Boolean array=w470) -> (number=w469:u32)
                n227 = case shown="2" w469 {
                  tunnel: w473 -> [_ w478 w484]
                  tunnel: w468 -> [_ _ w483]
                  tunnel: w467 -> [_ w477 _]
                  frame 0, Default {
                  }
                  frame 1 {
                    n228 = call "Sort Inductance Matrix.vi"("Current sorted?"=w477, "Inductance Matrix in"=w478) -> ("Inductance Matrix out"=w476:dbl[][])  [unwired: 2 in]
                    n229 = property on="Perm Magnet Flux Scalar" class="DigNum (strict)"("Visible"=FALSE) -> ()  [unwired: 2 in, 2 out]
                    n230 = property on="Permanent Magnet Flux (Fm)" class="Arr (strict)"("Visible"=TRUE) -> ()  [unwired: 2 in, 2 out]
                    n231 = local write "Permanent Magnet Flux (Fm)"(w476) -> ()
                  }
                  frame 2 {
                    n232 = call "Convert Fm to 2D array.vi"("Data in"=w484, "Data Cluster"=w483) -> ("Scalar data"=w482:dbl, "Data out"=w481:dbl[][])  [unwired: 7 in]
                    n233 = property on="Fm scalar" class="DigNum (strict)"("Visible"=TRUE) -> ()  [unwired: 2 in, 2 out]
                    n234 = local write "Permanent Magnet Flux (Fm)"(w481) -> ()
                    n235 = local write "Perm Magnet Flux Scalar"(w482) -> ()
                    n236 = property on="Fm 2D" class="Arr (strict)"("Visible"=FALSE) -> ()  [unwired: 2 in, 2 out]
                  }
                }
              }
            }
            n237 = call "Convert Unit (2D-Array).vi"("Data in"="Permanent Magnet Flux (Fm)", "unit"="Fm unit") -> ("Data out"=w458:dbl[][])  [unwired: 7 in]
            n238 = Bundle By Name(cluster=w456, "VDQ Model.Fm"=w458) -> (w464:T2)
            n239 = call-poly "Enqueue Message.vi"("error in (no error)"=w462, "Message"="Handle Tab Data", "Message Queue"=w460) -> ("error out"=w461:errorcluster)  [unwired: 7 in, 1 out]
          }
          frame 11 {
            n240 = call "Check Parameter Dimensions.vi"("Data Cluster"=w499) -> ("Size of Parameter arrays"=w493:T6, "Correct Dimension?"=w498:bool)  [unwired: 1 in]
            n241 = Unbundle(w493) -> ("Id size"=→"Id size":i32, "Iq size"=→"Iq size":i32, "Ld size"=→"Ld":i32[], "Lq size"=→"Lq":i32[], "FM size"=→"Fm":i32[])
            n242 = case shown="True" w498 {
              tunnel: w497 -> [w504 w511]
              tunnel: w496 -> [w505 w512]
              tunnel: [w503 w513] -> w487
              tunnel: ["The size of the Direct Current, Quadratic Current, Direct Inductance, Quadratic Inductance and Permanent Magnet Flux array do not match. \n- Direct Current array must be the same size as Quadratic Current array, and its values must be arranged in ascending order. - - Quadratic Current array must be the same size as Direct Current array, and its values must be arranged in ascending order. \n- Direct Inductance, Quadratic Inductance and Permanent Magnet Flux arrays must be n x n, where n is equal to the number of current values in Direct Current and Quadratic Current . \n" "The model data is ready to be converted into JSON file. The result file will be stored in the same folder of the reference spreadsheet file."] -> w495
              tunnel: [u32 16711680 ("Text.Text Colors:Text Color") u32 0 ("Text.Text Colors:Text Color")] -> w494
              tunnel: [w500 w507] -> _
              frame False {
                n243 = call-poly "Enqueue Message.vi"("error in (no error)"=w504, "Message"="Disable Convert", "Message Queue"=w505) -> ("error out"=w503:errorcluster, "dup Message Queue"=w500:refnum<queue>)  [unwired: 7 in]
              }
              frame True {
                n244 = call-poly "Enqueue Message.vi"("error in (no error)"=w511, "Message"="Enable Convert", "Message Queue"=w512) -> ("error out"=w513:errorcluster, "dup Message Queue"=w507:refnum<queue>)  [unwired: 7 in]
              }
            }
            "Status" <- w495
            n245 = property on="Status" class="Str"("Text.TextColor"=w494) -> ()  [unwired: 2 in, 2 out]
          }
          frame 12 {
            n246 = Unbundle By Name(w515) -> ("saved path"=→"JSON File Path":path)
            n247 = call-poly "Enqueue Message.vi"("error in (no error)"=w518, "Message"="Final UI State", "Message Queue"=w516) -> ("error out"=w517:errorcluster)  [unwired: 7 in, 1 out]
          }
        }
      }
      frame "Convert to JSON" {
        n248 = Unbundle By Name(w540) -> ("Active tab"=w537:u32, "selected path"=w542:path, "VDQ Model"=w529:T7)
        n249 = Increment(x=w537) -> (x+1=w530:u32)
        n250 = Unbundle By Name(w529) -> ("Ld"=w528:dbl[][], "Lq"=w526:dbl[][], "Fm"=w523:dbl[][])
        n251 = Transpose 2D Array(2D array=w526) -> (transposed array=w525:dbl[][])
        n252 = Transpose 2D Array(2D array=w523) -> (transposed array=w524:dbl[][])
        n253 = Transpose 2D Array(2D array=w528) -> (transposed array=w527:dbl[][])
        n254 = Empty String/Path?(string/path=w542) -> (empty?=w541:bool)
        n255 = Bundle By Name(cluster=w529, "Ld"=w527, "Lq"=w525, "Fm"=w524) -> (w522:T7)
        n256 = Flatten To JSON(anything=w522, error in (no error)=w521) -> (JSON string=w546:string, 11:w520:errorcluster)  [unwired: 1 in]
        n257 = case shown="False" w541 {
          tunnel: w542 -> [w557 _]
          tunnel: [w550 w558] -> w538
          frame False {
            n258 = Strip Path(path=w557) -> (stripped path=w556:path, name=w554:string)
            n259 = Match Pattern(string=w554, regular expression="[.]") -> (before substring=w553:string)  [unwired: 1 in, 3 out]
            n260 = Concatenate Strings(w553, ".json" ("string")) -> (w551:string)
            n261 = Build Path(base path=w556, name or relative path=w551) -> (appended path=w550:path)
          }
          frame True {
            n262 = call "File Dialog2"() -> ("selected path"=w558:path)  [unwired: 12 in, 3 out]
          }
        }
        n263 = call-poly "Enqueue Message.vi"("error in (no error)"=w520, "Message"="Update tab", "Message Queue"=w531) -> ("error out"=w532:errorcluster, "dup Message Queue"=w533:refnum<queue>)  [unwired: 7 in]
        n264 = call-poly "Enqueue Message.vi"("error in (no error)"=w532, "Message"="Handle Tab Data", "Message Queue"=w533) -> ("error out"=w536:errorcluster)  [unwired: 7 in, 1 out]
        n265 = Open/Create/Replace File(file path (use dialog)=w538, error in=w536, operation (0:open)=T5."replace or create") -> (refnum out=w548:refnum<file>, error out=w547:errorcluster)  [unwired: 3 in, 1 out]
        n266 = Bundle By Name(cluster=w540, "Active tab"=w530, "saved path"=w538) -> (w539:T2)
        n267 = Write to Text File(file (use dialog)=w548, text=w546, error in=w547) -> (refnum out=w545:refnum<file>, error out=w544:errorcluster)  [unwired: 1 in, 1 out]
        n268 = Close File(refnum=w545, error in=w544) -> (error out=w543:errorcluster)  [unwired: 1 out]
      }
      frame "Error" {
        # "#CodeRecommended - If you ever change the name of this \"Error\" message, you'll need to update the name in the Check Loop Error.vi as well."
        # "#CodeRecommended - Consider creating a system for logging errors in some way. These errors are for notification purposes only. Handling of specific errors should be performed in the message frames that generated the error."
        # "Error - Display an error dialog. This message is sent by the \"Error Handler\" VIs at the end of other loops in this application."
        n269 = Variant To Data(error in=w565, type=errorcluster {"status"=FALSE, "code"=0, "source"=""} ("error constant"), Variant=w563) -> (data=w561:errorcluster, error out=w560:errorcluster)
        n270 = call <vilib>:"Simple Error Handler.vi"("error in (no error)"=w561) -> ()  [unwired: 4 in, 5 out]
        n271 = Merge Errors(w560) -> (w559:errorcluster)
      }
      frame "Confirm Quit" {
        # "#CodeNeeded - If you want to provide an \"Are you sure\" dialog (or some other notification) before the application exits, place that code here. This message is typically sent from a Panel Close? event."
        # "Confirm Quit - Message that can confirm whether or not the user wants to exit the application."
        n272 = call-poly "Enqueue Message.vi"("Priority Message? (F)"=TRUE, "error in (no error)"=w572, "Message"="Exit", "Message Queue"=w568) -> ("error out"=w569:errorcluster)  [unwired: 6 in, 1 out]
        n273 = Merge Errors(w569) -> (w570:errorcluster)
      }
      frame "---Copy This Frame---" {
        # "Duplicate this frame when creating new messages.  Change this comment in the duplicated frame to describe this message."
        n274 = Merge Errors(w575) -> (w573:errorcluster)
      }
      frame "Exit" {
        # "Stop the VI"
        # "Release the message queue reference"
        # "#CodeNeeded - Add any required cleanup code here. Note that if 'Exit' was called as a result of an error, an error dialog will be displayed. Add any custom error handling for an 'Exit' condition here as well."
        # "Exit - Exit the application."
        n275 = Variant To Data(type=errorcluster {"status"=FALSE, "code"=0, "source"=""} ("error constant"), Variant=w576) -> (data=w577:errorcluster)  [unwired: 1 in, 1 out]
        n276 = call <vilib>:"Simple Error Handler.vi"("error in (no error)"=w577) -> ()  [unwired: 4 in, 5 out]
        n277 = call "Fire User Event - Stop.vi"("User Event - Stop"=w581) -> ("error out"=w580:errorcluster)  [unwired: 10 in]
        n278 = Release Queue(queue=w586, error in (no error)=w579) -> (error out=w583:errorcluster)  [unwired: 1 in, 2 out]
        n279 = Merge Errors(w580, w583) -> (w582:errorcluster)
      }
      frame Default {
        # "'Default' case only runs if there is a message that isn't defined in any of the other cases.  Output a programming error."
        n280 = xnode "Error Ring"("parameter 0"=w587) -> ("error out"=w588:errorcluster)
      }
    }
    n281 = call "Error Handler - Message Handling Loop.vi"("error in (no error)"=w16, "Message Queue"=w18) -> ("dup error in"=w17:errorcluster)  [unwired: 8 in, 1 out]
  }
  n282 = while {
    tunnel: w12 -> [w603]
    shift-right: [w601] -> w8
    shift-left: w4 -> [w602]
    tunnel: [w597] -> w5
    stop <- w599 stop-if-true
    # "Event Handling Loop"
    n283 = event shown="[6] \"Perm Magnet Flux Scalar\": Value Change" {
      selector: w602 -> [_ _ _ _ _ _ _ _ _ _]
      dyn-events: [_ _ _ _ _ _ _ _ _ _] -> w601
      timeout: _ -> [_ _ _ _ _ _ _ _ _ _]
      tunnel: [_ _ _ _ _ _ _ _ _ TRUE ("Discard?")] -> w599
      tunnel: w603 -> [w610 w613 w620 w624 w628 w631 w635 w643 w645 w647]
      tunnel: [w605 w611 w618 w622 w626 w632 w636 w642 _ _] -> w600
      tunnel: [w604 w612 w619 w623 w627 w630 w637 w641 w645 w647] -> w598
      event "Next": Value Change {
        n284 = event-data() -> ()  [unwired: 1 in, 1 out]
        n285 = call-poly "Enqueue Message.vi"("Message"="Next tab", "Message Queue"=w610) -> ("error out"=w606:errorcluster, "dup Message Queue"=w607:refnum<queue>)  [unwired: 8 in]
        n286 = call-poly "Enqueue Message.vi"("error in (no error)"=w606, "Message"="Handle Tab Data", "Message Queue"=w607) -> ("error out"=w605:errorcluster, "dup Message Queue"=w604:refnum<queue>)  [unwired: 7 in]
      }
      event "Back": Value Change {
        n287 = event-data() -> ()  [unwired: 1 in, 1 out]
        n288 = call-poly "Enqueue Message.vi"("Message"="Previous tab", "Message Queue"=w613) -> ("error out"=w614:errorcluster, "dup Message Queue"=w615:refnum<queue>)  [unwired: 8 in]
        n289 = call-poly "Enqueue Message.vi"("error in (no error)"=w614, "Message"="Handle Tab Data", "Message Queue"=w615) -> ("error out"=w611:errorcluster, "dup Message Queue"=w612:refnum<queue>)  [unwired: 7 in]
      }
      event "Convert": Value Change {
        n290 = event-data() -> ()  [unwired: 1 in, 1 out]
        n291 = call-poly "Enqueue Message.vi"("Message"="Convert to JSON", "Message Queue"=w620) -> ("error out"=w618:errorcluster, "dup Message Queue"=w619:refnum<queue>)  [unwired: 8 in]
      }
      event "Restart": Value Change {
        n292 = event-data() -> ()  [unwired: 1 in, 1 out]
        n293 = call-poly "Enqueue Message.vi"("Message"="Initialize", "Message Queue"=w624) -> ("error out"=w622:errorcluster, "dup Message Queue"=w623:refnum<queue>)  [unwired: 8 in]
      }
      event "Finish": Value Change {
        n294 = event-data() -> ()  [unwired: 1 in, 1 out]
        n295 = call-poly "Enqueue Message.vi"("Message"="Exit", "Message Queue"=w628) -> ("error out"=w626:errorcluster, "dup Message Queue"=w627:refnum<queue>)  [unwired: 8 in]
      }
      event "Load File": Value Change {
        n296 = event-data() -> ()  [unwired: 1 in, 1 out]
        n297 = call-poly "Enqueue Message.vi"("Message"="Open file", "Message Queue"=w631) -> ("error out"=w632:errorcluster, "dup Message Queue"=w630:refnum<queue>)  [unwired: 8 in]
      }
      event "Perm Magnet Flux Scalar": Value Change {
        n298 = event-data() -> ()  [unwired: 1 in, 1 out]
        n299 = call-poly "Enqueue Message.vi"("Message Data"="Perm Magnet Flux Scalar", "Message"="Scalar Fm", "Message Queue"=w635) -> ("error out"=w636:errorcluster, "dup Message Queue"=w637:refnum<queue>)  [unwired: 7 in]
      }
      event Panel Close? {
        # "Send the 'Confirm Quit' message if the user closes the panel of the VI. Discard the event so the 'Confirm Quit' message has a chance to run."
        n300 = event-data() -> ()  [unwired: 1 in, 1 out]
        n301 = call-poly "Enqueue Message.vi"("Priority Message? (F)"=TRUE, "Message"="Confirm Quit", "Message Queue"=w643) -> ("error out"=w642:errorcluster, "dup Message Queue"=w641:refnum<queue>)  [unwired: 7 in]
        n302 = event-data("Discard?"=TRUE) -> ()  [unwired: 1 in, 1 out]
      }
      event Application Instance Close {
        # "#CodeRecommended - When a project closes, all VIs within that project are aborted and leave memory. However, any code placed in this event frame is guaranteed to run to completion, so add any cleanup code that absolutely must happen here."
        n303 = event-data() -> ()  [unwired: 1 in, 1 out]
      }
      event User Event {
        # "The Message Handling Loop processed an \"Exit\" message, which fired this event to stop the Event Handling Loop."
        n304 = event-data() -> ()  [unwired: 1 in, 1 out]
      }
    }
    n305 = call "Error Handler - Event Handling Loop.vi"("error in (no error)"=w600, "Message Queue"=w598) -> ("dup error in"=w597:errorcluster)  [unwired: 8 in, 1 out]
  }
  n306 = Unregister For Events(event registration refnum=w8, error in=w5) -> (error out=w9:errorcluster)
  n307 = Merge Errors(w9, w13) -> (w10:errorcluster)
  n308 = call "Destroy User Event - Stop.vi"("error in (no error)"=w10, "User Event - Stop"=w3) -> ("error out"=w6:errorcluster)  [unwired: 9 in]
  n309 = disable-structure shown="RUN_TIME_ENGINE==True" {
    disable-tunnel: w6 -> [_ _]
    frame condition #0 (active) {
    }
    frame condition #1 {
      # "Call Quit LabVIEW if running as a built application."
      n310 = Quit LabVIEW() -> ()  [unwired: 1 in]
    }
  }
